vi "RVC 3-link serial robot Scara.vi"() -> ()   [LabVIEW 2014]
uses:
  <vilib>/Analysis/Matrix/Datatypes/RealMatrix.ctl
  <vilib>/robotics/Kinematics/Analytical/Initialize Generic Serial Arm.vi
  <vilib>/robotics/Kinematics/Analytical/NI_Robotics_AnalyticKinematics.lvlib
  <vilib>/robotics/Kinematics/Robot/NI_Robotics_Serial Robot Arm.lvclass
  <vilib>/Analysis/Matrix/NI_Matrix.lvlib
panel:
  in  "appended array":dbl[](array[numeric])=[0.6, -1.0, 0.3, 0.0]
  out "transformation":picture
  out "forward kinematics":T1
  out "3D Picture":refnum<vi>(3d-picture)
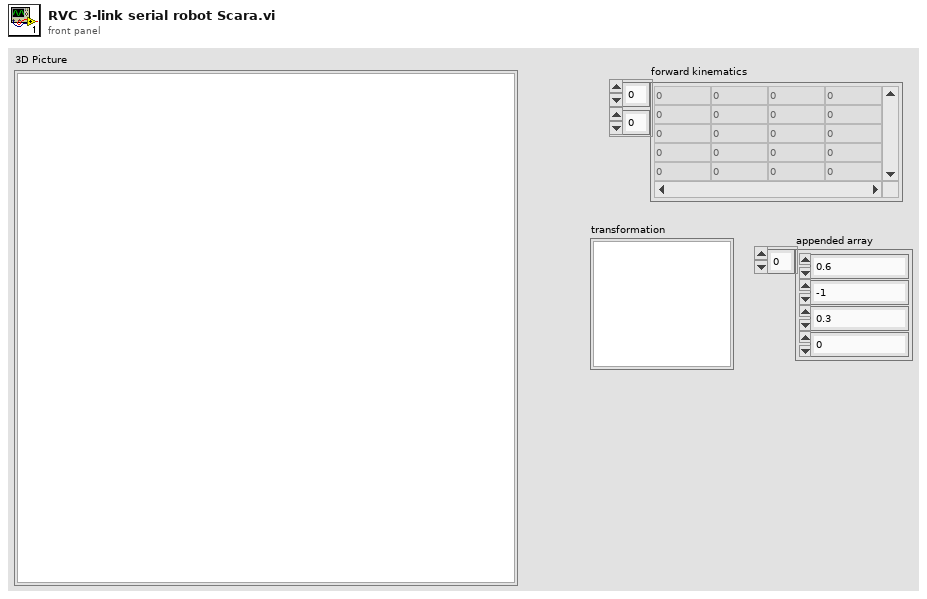
[diagram p1: front panel]
types:
  T1 = typedef "NI_Matrix.lvlib/RealMatrix.ctl" = dbl[][]
  T2 = typedef "DH Kinematic Parameters.ctl" = cluster{"twist angle":dbl, "length":dbl, "rotation angle":dbl, "offset distance":dbl, "joint type":T3, "joint coordinate offset":dbl}
  T3 = typedef "NI_Robotics_Link.lvclass/Joint Type.ctl" = enum16{"Revolute", "Prismatic"}
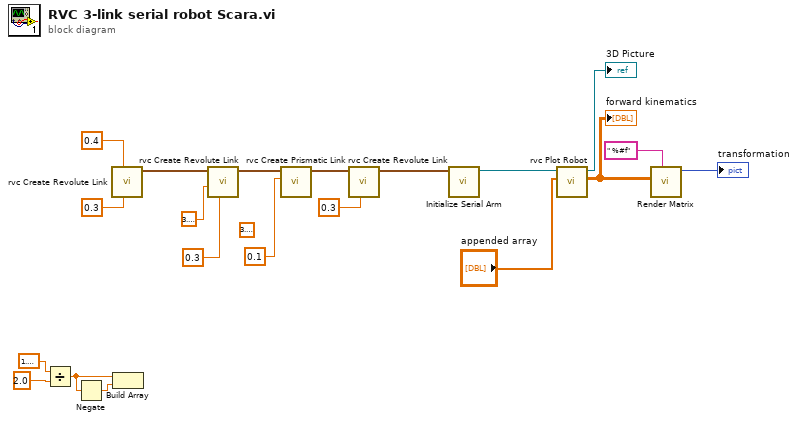
[diagram p0: block diagram]
diagram:
  (unwired) 3.141592653589793
  n1 = Divide(x=1.5707963267948966, y=2.0) -> (x/y=w16:dbl)
  n2 = Negate(x=w16) -> (-x=w15:dbl)
  n3 = call "rvc Create Revolute Link.vi"("length (a)"=0.3, "offset distance (d)"=0.4) -> ("Array"=w9:T2[])  [unwired: 9 in]
  n4 = Build Array(w16, w15) -> ()  [unwired: 1 out]
  n5 = call "rvc Create Revolute Link.vi"("length (a)"=0.3, "twist angle (alpha)"=3.141592653589793, "Array 2"=w9) -> ("Array"=w10:T2[])  [unwired: 8 in]
  n6 = call "rvc Create Prismatic Link.vi"("length (a)"=0.1, "Array 2"=w10) -> ("Array"=w4:T2[])  [unwired: 9 in]
  n7 = call "rvc Create Revolute Link.vi"("length (a)"=0.3, "Array 2"=w4) -> ("Array"=w3:T2[])  [unwired: 9 in]
  n8 = call-poly <vilib>:"Initialize Serial Arm.vi"("kinematic parameters"=w3) -> ("serial arm out"=w20:refnum<class "NI_Robotics_Serial Robot Arm.lvclass">)  [unwired: 9 in, 1 out]
  n9 = call "rvc Plot Robot.vi"("joint positions"="appended array", "NI_Robotics_Serial Robot Arm in"=w20) -> ("forward kinematics"=w12:T1, "Scene Object Out"=→"3D Picture":refnum<vi>)  [unwired: 7 in, 1 out]
  "forward kinematics" <- w12
  n10 = call "Render Matrix.vi"("format string"=" %#f", "A"=w12) -> ("picture out"=→"transformation":picture)  [unwired: 9 in]
